vi "MakeColHeaderString.vi"(11 "CH名称(複数行)":string[][](array[string])) -> (3 "CH名称(1行)":string[](array[string]))   [LabVIEW 2014]
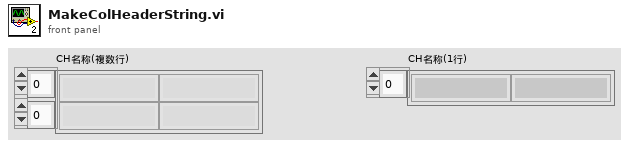
[diagram p1: front panel]
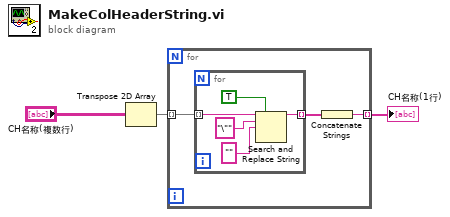
[diagram p0: block diagram]
diagram:
  n1 = Transpose 2D Array(2D array="CH名称(複数行)") -> (transposed array=w1:string[][])
  n2 = for {
    tunnel: w1 -> [w6] mode=indexing
    tunnel: [w4] -> w3 mode=indexing
    n3 = for {
      tunnel: w6 -> [w11] mode=indexing
      tunnel: [w7] -> w5 mode=indexing
      n4 = Search and Replace String(replace all?=TRUE ("すべて置換?(F)"), input string=w11, search string="\"" ("検索文字列"), replace string="" ("置換文字列（\"\"）")) -> (result string=w7:string)  [unwired: 4 in, 3 out]
    }
    n5 = Concatenate Strings(w5) -> (w4:string)
  }
  "CH名称(1行)" <- w3
